vi "VMI_analyse_refs_remove.vi"(0 "Peak Position Queue in":T1, 1 "Test Timing":bool, 2 "Image Options":refnum<vi>, 5 "Image Control Reference":refnum<vi>, 9 "Image in":T1, 11 "Stop Button Ref":refnum<vi>, 12 "Image_array":i32[][](array[numeric]), 14 "Acquire Time":i32) -> (3 "Image_array out":i32[][](array[numeric]), 4 "Peaks Position Out":cluster{"X":sgl, "Y":sgl}[](array[cluster]), 6 "Current Image":T2(plugin-control), 10 "Peaks per frame":i32[](array[numeric]), 15 "error out":errorcluster)   [LabVIEW 2019]
uses:
  <vilib>/vision/Image Controls.llb/IMAQ Image.ctl
panel:
  out "x-y":u32
  out "size(s)":i32
  out "Single Image Points":cluster{"X":sgl, "Y":sgl}[](array[cluster])=[{"X"=212.6804, "Y"=106.63919}, {"X"=138.40689, "Y"=24.241379}, {"X"=316.33078, "Y"=38.515385}, {"X"=320.0, "Y"=56.301075}, {"X"=193.84746, "Y"=79.23729}, {"X"=195.92592, "Y"=104.85185}, {"X"=101.513275, "Y"=109.92921}, {"X"=345.82178, "Y"=117.28713}, {"X"=240.13792, "Y"=145.94827}, {"X"=10.357142, "Y"=157.24026}, {"X"=232.16667, "Y"=157.69608}, {"X"=104.34286, "Y"=174.28572}, {"X"=15.540541, "Y"=195.72298}, {"X"=93.1018, "Y"=207.8024}, {"X"=230.61539, "Y"=255.9011}, {"X"=129.26056, "Y"=275.0845}, {"X"=109.85714, "Y"=276.10715}, {"X"=46.11494, "Y"=281.16092}, {"X"=157.0, "Y"=298.7595}, {"X"=134.89635, "Y"=321.72562}]
  in  "Stop Button":bool
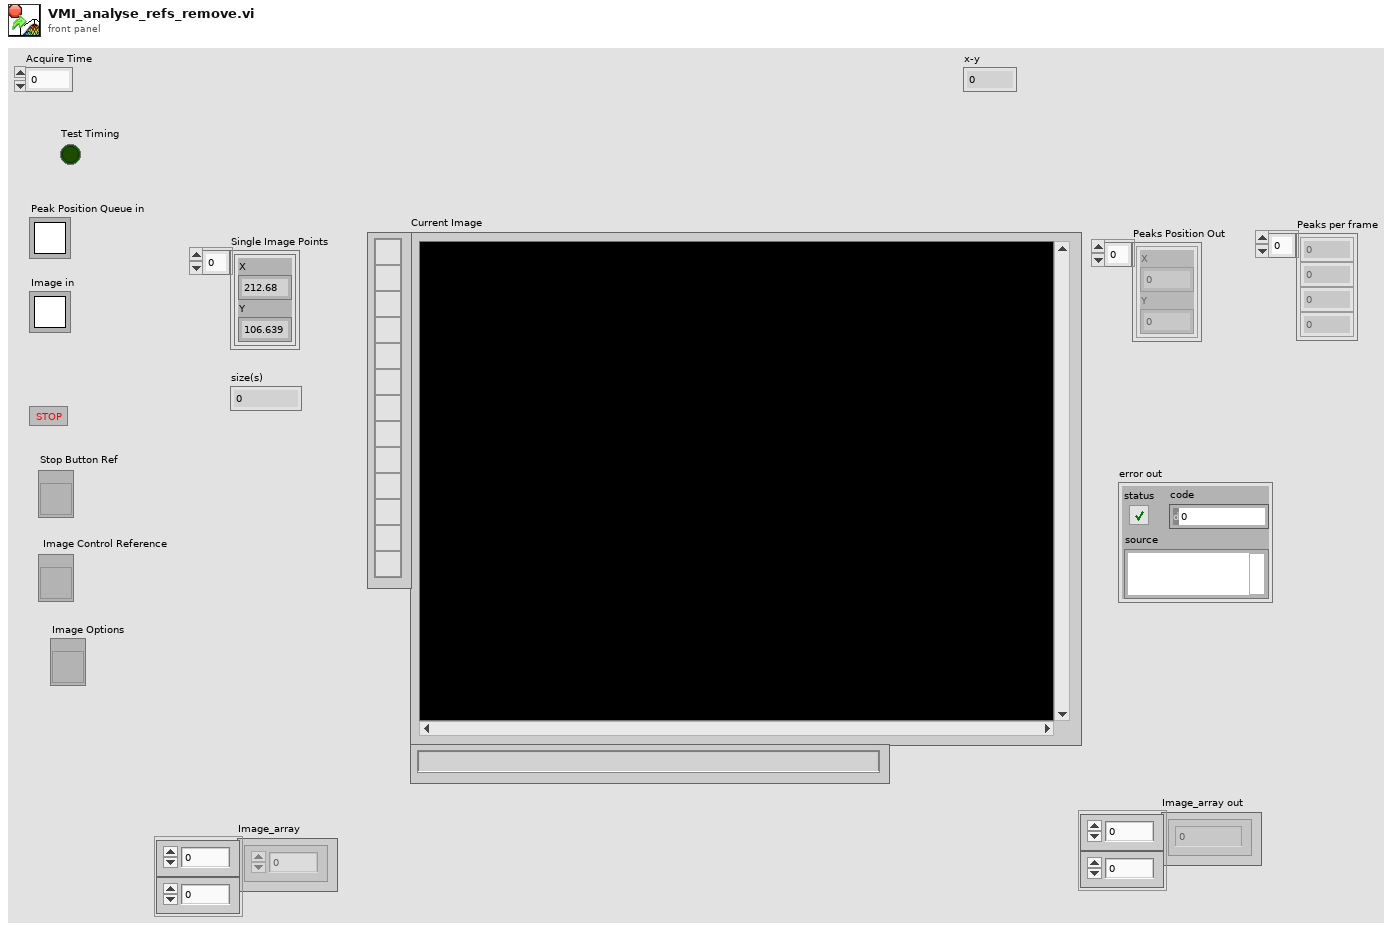
[diagram p1: front panel]
types:
  T1 = typedef "Queue RefNum" = refnum<k1>
  T2 = typedef "IMAQ Image.ctl" = refnum<image>
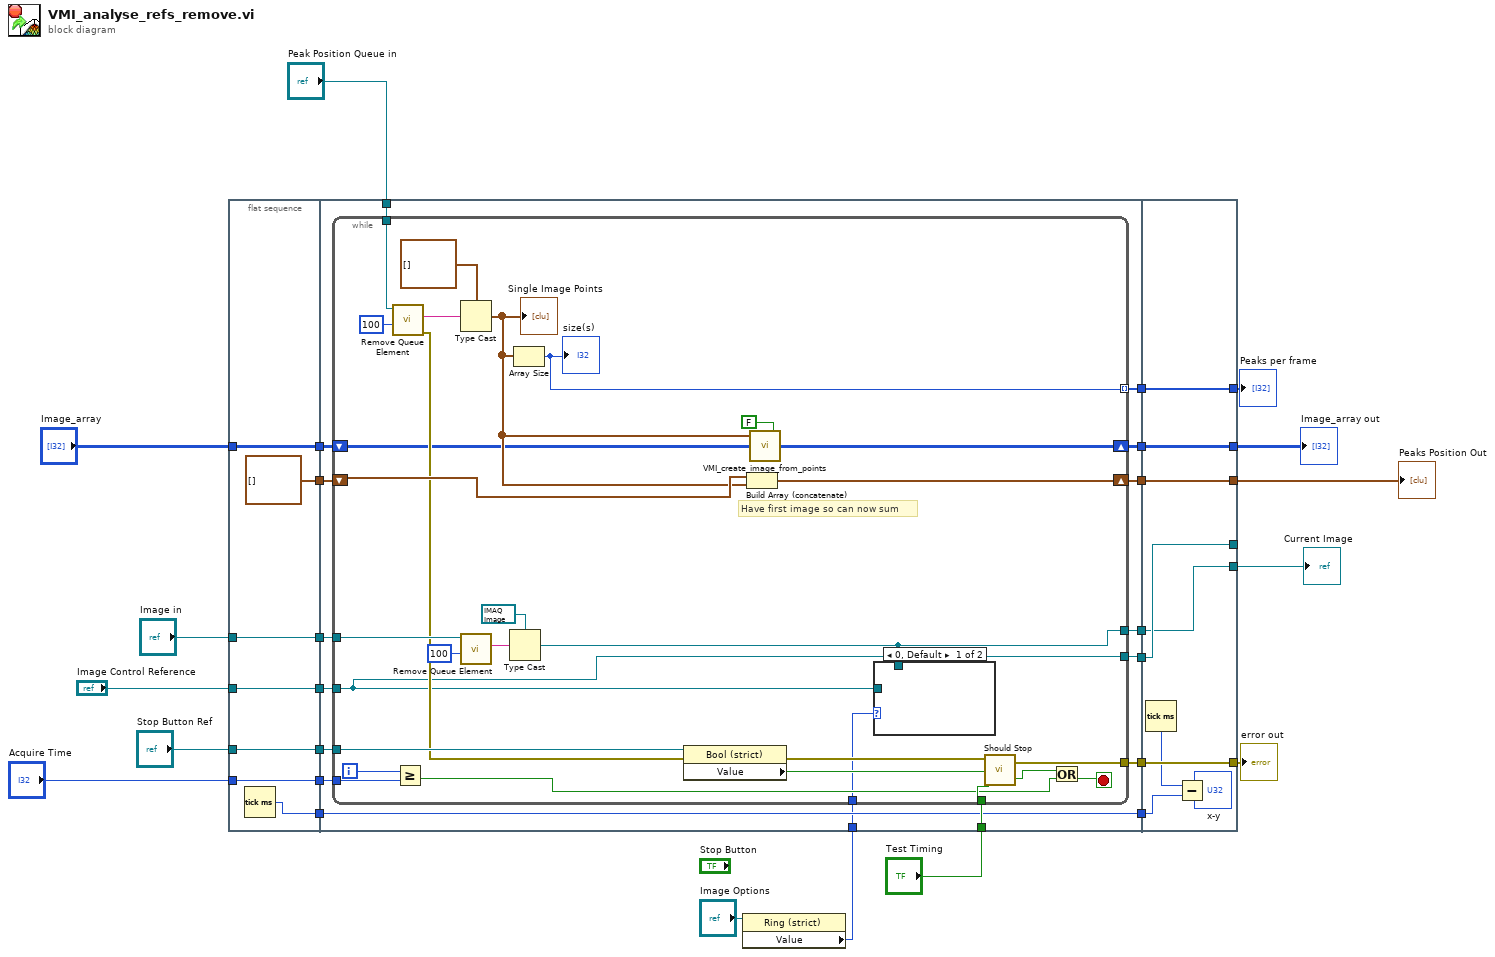
[diagram p0: block diagram]
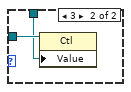
[diagram p2: hidden frame]
diagram:
  n1 = flat-sequence {
    tunnel: "Acquire Time" -> [w33]
    tunnel: "Stop Button Ref" -> [w34]
    tunnel: "Image in" -> [w35]
    tunnel: [w35] -> w17
    tunnel: [w34] -> w16
    tunnel: [w33] -> w15
    tunnel: [w32] -> w13
    tunnel: "Image Control Reference" -> [w31]
    tunnel: [w31] -> w11
    tunnel: [cluster{"X":sgl, "Y":sgl}[] []] -> w5
    tunnel: "Image_array" -> [w29]
    tunnel: [w29] -> w3
    tunnel: "Peak Position Queue in" -> [w49]
    tunnel: "Test Timing" -> [w46]
    tunnel: [w51] -> w20
    tunnel: [w48] -> w19
    tunnel: [w47] -> w18
    tunnel: w17 -> [w50]
    tunnel: w16 -> [w45]
    tunnel: w15 -> [w44]
    tunnel: [w43] -> w14
    tunnel: w13 -> [w43]
    tunnel: w11 -> [w42]
    tunnel: w9 -> [w41]
    tunnel: [w40] -> w8
    tunnel: [w39] -> w7
    tunnel: w5 -> [w38]
    tunnel: [w37] -> w4
    tunnel: w3 -> [w36]
    tunnel: [w89] -> w24
    tunnel: [w90] -> w25
    tunnel: [w91] -> w28
    tunnel: w20 -> [w91]
    tunnel: w19 -> [w90]
    tunnel: w18 -> [w89]
    tunnel: w14 -> [w88]
    tunnel: w8 -> [w85]
    tunnel: [w85] -> _
    tunnel: w7 -> [w84]
    tunnel: [w84] -> w6
    tunnel: w4 -> [w83]
    tunnel: [w83] -> w1
    frame #0 {
      n2 = Tick Count (ms)() -> (millisecond timer value=w32:u32)
    }
    frame #1 {
      n3 = while {
        tunnel: w49 -> [w80]
        tunnel: w50 -> [w77]
        shift-right: [w74] -> w48
        shift-left: w38 -> [w73]
        tunnel: [w72] -> w51
        tunnel: [w71] -> w47 mode=indexing
        tunnel: w46 -> [w70]
        tunnel: w45 -> [w69]
        tunnel: w44 -> [w64]
        tunnel: [w58] -> w39
        tunnel: w42 -> [w56]
        tunnel: w41 -> [w57]
        tunnel: [w56] -> w40
        shift-right: [w54] -> w37
        shift-left: w36 -> [w53]
        i -> [w65]
        stop <- w63 stop-if-true
        # "Have first image so can now sum"
        n4 = call <vilib>:"Remove Queue Element.vi"("ms timeout (-1)"=100, "queue"=w80) -> ("error out"=w67:errorcluster, "queue element"=w79:string)  [unwired: 4 in, 2 out]
        n5 = Greater Or Equal?(x=w65, y=w64) -> (x >= y?=w61:bool)
        n6 = Type Cast(type=cluster{"X":sgl, "Y":sgl}[] [], x=w79) -> (*(type *) &x=w55:cluster{"X":sgl, "Y":sgl}[])
        "Single Image Points" <- w55
        n7 = call <vilib>:"Remove Queue Element.vi"("ms timeout (-1)"=100, "queue"=w77) -> ("queue element"=w76:string)  [unwired: 4 in, 3 out]
        n8 = Type Cast(type=T2 refnum ("Image Out"), x=w76) -> (*(type *) &x=w58:T2)
        n9 = Array Size(array=w55) -> (size(s)=w71:i32)
        "size(s)" <- w71
        n10 = property class="Bool (strict)"(reference=w69, error in=w67) -> (error out=w66:errorcluster, "Value"=w68:bool)  [unwired: 1 out]
        n11 = Build Array (concatenate)(w73, w55) -> (w74:cluster{"X":sgl, "Y":sgl}[])
        n12 = call "VMI_create_image_from_points.vi"("New Array"=FALSE, "Input array"=w53, "Points"=w55) -> ("Image Array"=w54:i16[][])  [unwired: 2 in]
        n13 = case shown="0, Default" w57 {
          tunnel: w56 -> [_ w82]
          tunnel: w58 -> [_ w81]
          frame 0, Default {
          }
          frame 3 {
            n14 = property class="Ctl"(reference=w82, "Value"=w81) -> ()  [unwired: 1 in, 2 out]
          }
        }
        n15 = call "Should Stop.vi"("error in 1"=w66, "Stop Button"=w68, "Look at Stop Button"=w70) -> ("error out"=w72:errorcluster, "Stop"=w62:bool)  [unwired: 2 in]
        n16 = Or(x=w62, y=w61) -> (x .or. y?=w63:bool)
      }
    }
    frame #2 {
      n17 = Tick Count (ms)() -> (millisecond timer value=w87:u32)
      n18 = Subtract(x=w87, y=w88) -> (x-y=→"x-y":u32)
    }
  }
  n19 = property class="Ring (strict)"(reference="Image Options") -> ("Value"=w9:u16)  [unwired: 1 in, 2 out]
  "error out" <- w28
  "Peaks Position Out" <- w25
  "Current Image" <- w6
  "Peaks per frame" <- w24
  "Image_array out" <- w1
